vi "Add Points to Series_DBL.vi"(6 "YValuesPerPoint":i32=1, 8 "error in (no error)":errorcluster, 9 "Data":dbl[](array[numeric]), 10 ".NET MSChart Series":refnum<k24>) -> (0 "error out":errorcluster, 2 ".NET MSChart Series (dup)":refnum<k24>)   [LabVIEW 2014, in "XMSChart.xctl"]
uses:
  XMSChart.xctl
  System.Windows.Forms.DataVisualization
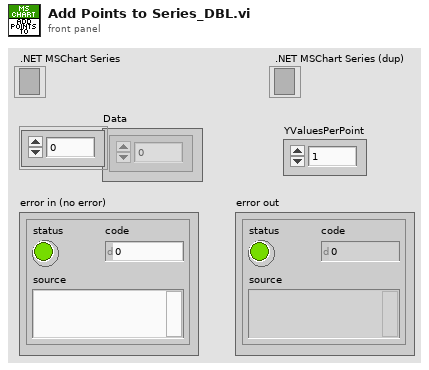
[diagram p1: front panel]
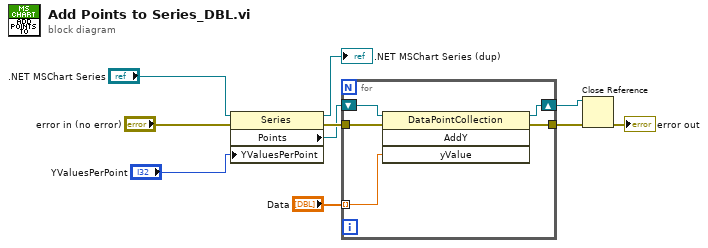
[diagram p0: block diagram]
diagram:
  n1 = property on="Property Node" class="Series"(reference=".NET MSChart Series", error in="error in (no error)", "YValuesPerPoint"="YValuesPerPoint") -> (reference out=→".NET MSChart Series (dup)":refnum<k24>, error out=w7:errorcluster, "Points"=w6:refnum<k24>)
  n2 = for {
    tunnel: "Data" -> [w14] mode=indexing
    tunnel: [w12] -> w2
    shift-right: [w13] -> w4
    shift-left: w6 -> [w15]
    tunnel: w7 -> [w11]
    n3 = invoke class="DataPointCollection" method="AddY"(reference=w15, error in=w11, "yValue"=w14) -> (reference out=w13:refnum<k24>, error out=w12:errorcluster)  [unwired: 1 in, 2 out]
  }
  n4 = Close Reference(reference=w4, error in (no error)=w2) -> (error out=→"error out":errorcluster)
